vi "Parse.vi"(8 "error in (no error)":errorcluster, 10 "Transfer Group in":refnum<class "Transfer Group.lvclass">, 11 "Type Converter in":refnum<class "Simple Type Converter.lvclass">) -> (0 "error out":errorcluster, 2 "Transfer Group out":refnum<class "Transfer Group.lvclass">, 3 "Type Converter out":refnum<class "Simple Type Converter.lvclass">)   [LabVIEW 2017, in "DSF Core.lvlib" / "Simple Type Converter.lvclass"]
uses:
  Simple Type Converter.lvclass
  Classes/Transfer Group/Transfer Group.lvclass
  Simple Type Converter.lvclass/Simple Type Converter.ctl
  Convert String Block.vi
  Classes/Buffer/Read Buffer 1D U8.vi
  VIs/Sizeof 1D.vi
  Classes/Buffer/Write Buffer 1D U8.vi
  Classes/Buffer/Buffer.lvclass
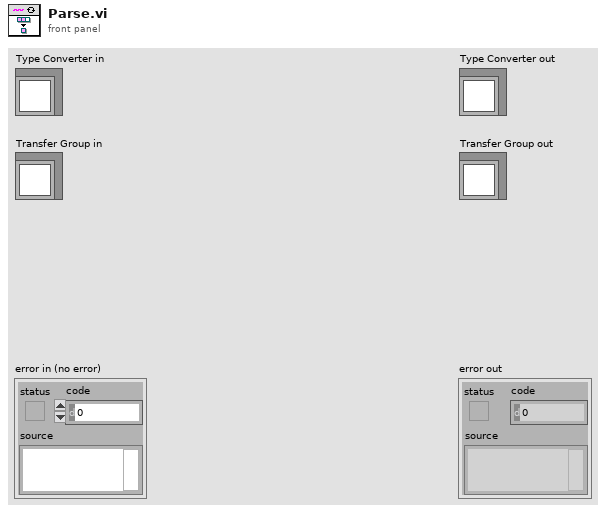
[diagram p1: front panel]
types:
  T1 = typedef "DSF Core.lvlib/Simple Type Converter.lvclass/Conversion.ctl" = cluster{"conversion blocks":T2[]}
  T2 = typedef "DSF Core.lvlib/Simple Type Converter.lvclass/Conversion Block.ctl" = cluster{"engine offset":u64, "engine data type":T3, "string offset":u64, "string data type":T3, "engine byte order":enum16{"big-endian, network order", "native, host order", "little-endian"}, "string byte order":enum16{"big-endian, network order", "native, host order", "little-endian"}, "count":u64}
  T3 = typedef "DSF Core.lvlib/DSF Data Type.ctl" = enum8{"Bool", "SGL", "DBL", "I8", "I16", "I32", "I64", "U8", "U16", "U32", "U64"}
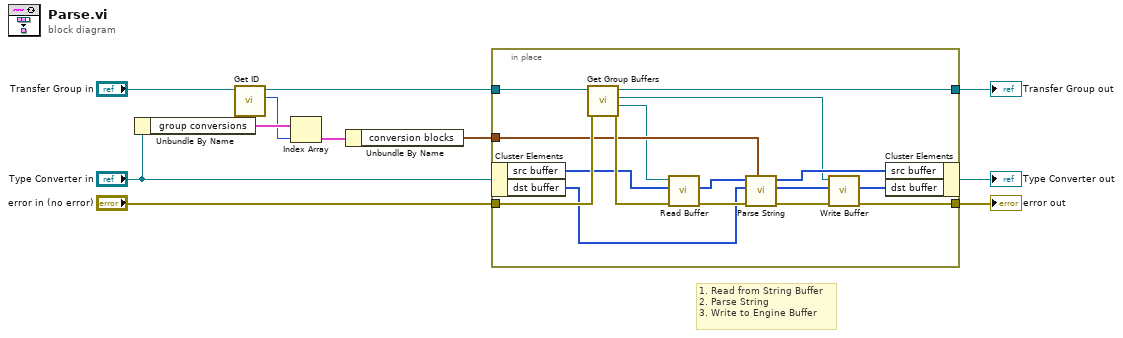
[diagram p0: block diagram]
diagram:
  # "1. Read from String Buffer\n2. Parse String\n3. Write to Engine Buffer"
  n1 = Unbundle By Name("Type Converter in") -> ("group conversions"=w11:T1[])
  n2 = call "Get ID.vi"("Transfer Group in"="Transfer Group in") -> ("id"=w8:i32, "Transfer Group out"=w7:refnum<class "Transfer Group.lvclass">)  [unwired: 9 in]
  n3 = Index Array(array=w11, index=w8) -> (element=w10:T1)
  n4 = Unbundle By Name(w10) -> ("conversion blocks"=w9:T2[])
  n5 = in-place {
    in-place-border: w9 -> [w18]
    in-place-border: [w24] -> w4
    in-place-border: "error in (no error)" -> [w23]
    in-place-border: w7 -> [w22]
    in-place-border: [w19] -> w1
    n6 = in-place-cluster #1("Type Converter in") -> ("src buffer"=w15:u8[], "dst buffer"=w20:u8[])
    n7 = call "Get Group Buffers.vi"("error in (no error)"=w23, "Transfer Group in"=w22) -> ("error out"=w21:errorcluster, "string Buffer"=w17:refnum<class "Buffer.lvclass">, "engine Buffer"=w16:refnum<class "Buffer.lvclass">, "Transfer Group out"=w19:refnum<class "Transfer Group.lvclass">)  [unwired: 6 in]
    n8 = call-poly "Read Buffer.vi"("error in (no error)"=w21, "dst array in"=w15, "Buffer in"=w17) -> ("error out"=w26:errorcluster, "dst array out"=w14:u8[])  [unwired: 5 in, 2 out]
    n9 = call "Parse String.vi"("conversion blocks"=w18, "error in (no error)"=w26, "dst buffer in"=w20, "src buffer in"=w14) -> ("error out"=w25:errorcluster, "dst buffer out"=w12:u8[], "src buffer out"=w27:u8[])  [unwired: 5 in]
    n10 = call-poly "Write Buffer.vi"("error in (no error)"=w25, "src array in"=w12, "Buffer in"=w16) -> ("error out"=w24:errorcluster, "src array out"=w13:u8[])  [unwired: 5 in, 2 out]
    n11 = in-place-cluster #1("src buffer"=w27, "dst buffer"=w13) -> (→"Type Converter out":refnum<class "Simple Type Converter.lvclass">)
  }
  "error out" <- w4
  "Transfer Group out" <- w1
